vi "Joystick Scaling.vi"(2 "Scale (%)":dbl=100.0 min=0.0 max=100.0 step=1.0, 3 "Input (+/- 1.00 volt)":dbl(slide) scale=-1.0..1.0) -> (0 "Output":dbl)   [LabVIEW 2012]
panel:
  # "Slew rate limiting limits the effective rate at which the motors may accelerate by only allowing the signal to change by a small fixed amount each time the code executes."
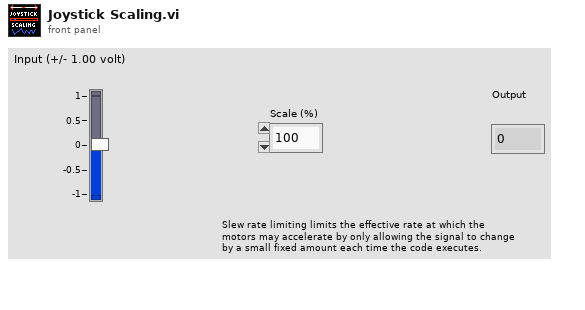
[diagram p1: front panel]
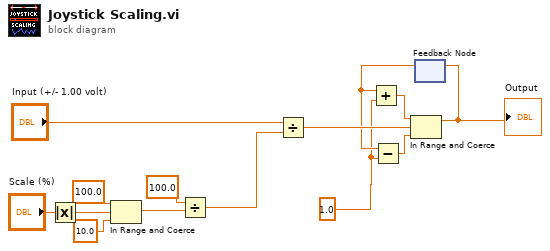
[diagram p0: block diagram]
diagram:
  w1 = 1.0 ("y")
  n1 = Absolute Value(x="Scale (%)") -> (abs(x)=w6:dbl)
  n2 = In Range and Coerce(upper limit=100.0, x=w6, lower limit=10.0) -> (coerced(x)=w12:dbl)  [unwired: 1 out]
  n3 = Divide(x=100.0, y=w12) -> (x/y=w8:dbl)
  n4 = Divide(x="Input (+/- 1.00 volt)", y=w8) -> (x/y=w14:dbl)
  n5 = feedback #1() -> (w2:dbl)  [unwired: 1 in]
  n6 = Add(x=w2, y=w1) -> (x+y=w5:dbl)
  n7 = Subtract(x=w2, y=w1) -> (x-y=w4:dbl)
  n8 = In Range and Coerce(upper limit=w5, x=w14, lower limit=w4) -> (coerced(x)=w3:dbl)  [unwired: 1 out]
  "Output" <- w3
  n9 = feedback-in #1(w3) -> ()
